vi "loadProg.vi"(11 "selected path":path) -> (0 "error out":errorcluster, 2 "scenes":T1[](array[typedef]), 3 "editArray":T2[](array[typedef]))   [LabVIEW 2014]
uses:
  typeDefs/editControl.ctl
  typeDefs/variantFlat.ctl
  typeDefs/pictChooser.ctl
  typeDefs/saveDataType.ctl
  <vilib>/picture/picture.llb/Draw True-Color Pixmap.vi
  <vilib>/Utility/config.llb/NI_LVConfig.lvlib
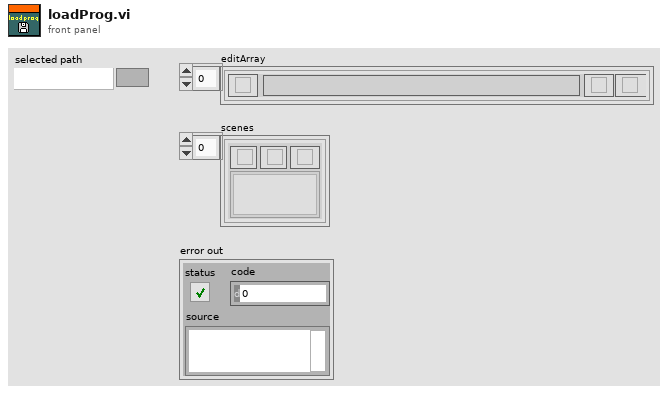
[diagram p1: front panel]
types:
  T1 = typedef "pictChooser.ctl" = cluster{"2D Picture":picture, "load":bool, "Path":path, "Bitmap":u32[][], "del":bool, "paint":bool}
  T2 = typedef "editControl.ctl" = cluster{"edit":bool, "info":string, "variantFlat":T3, "codeCluster":cluster{"code":u8[][]}, "del":bool, "ins":bool}
  T3 = typedef "variantFlat.ctl" = cluster{"type string":i16[], "data string":string}
  T4 = typedef "saveDataType.ctl" = cluster{"editArray":T2[], "bitmaps":cluster{"Bitmap":u32[][]}[], "paths":path[]}
  T5 = typedef "NI_LVConfig.lvlib/Config Data RefNum.ctl" = refnum<k1>
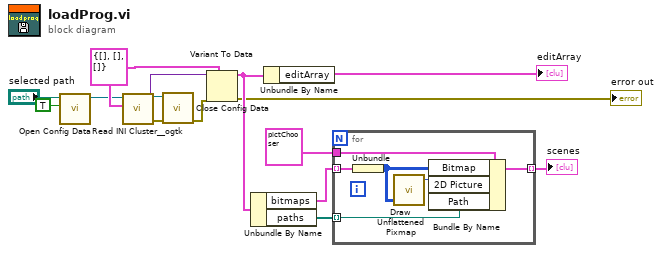
[diagram p0: block diagram]
diagram:
  w9 = T4 {"editArray"=[], "bitmaps"=[], "paths"=[]} ("saveData")
  n1 = call <vilib>:"Open Config Data.vi"("create file if necessary (T)"=TRUE, "configuration file path"="selected path") -> ("refnum"=w3:T5)  [unwired: 7 in, 2 out]
  n2 = call <userlib>:"Read INI Cluster__ogtk.vi"("INI Fomatted Cluster Type"=w9, "refnum"=w3) -> ("error out"=w4:errorcluster, "INI Fomatted Cluster"=w6:variant, "dup refnum"=w5:T5)  [unwired: 5 in, 2 out]
  n3 = call <vilib>:"Close Config Data.vi"("error in (no error)"=w4, "refnum"=w5) -> ("error out"=w7:errorcluster)  [unwired: 8 in, 1 out]
  n4 = Variant To Data(error in=w7, type=w9, Variant=w6) -> (data=w10:T4, error out=→"error out":errorcluster)
  n5 = Unbundle By Name(w10) -> ("bitmaps"=w11:cluster{"Bitmap":u32[][]}[], "paths"=w14:path[])
  n6 = Unbundle By Name(w10) -> ("editArray"=→"editArray":T2[])
  n7 = for {
    tunnel: w11 -> [w21] mode=indexing
    tunnel: T1 {"2D Picture"=bytes[0], "load"=FALSE, "Path"=path "", "Bitmap"=[], "del"=FALSE, "paint"=FALSE} ("pictChooser") -> [w20]
    tunnel: [w19] -> w13 mode=indexing
    tunnel: w14 -> [w16] mode=indexing
    n8 = Unbundle(w21) -> ("Bitmap"=w17:u32[][])
    n9 = call-poly <vilib>:"Draw Unflattened Pixmap.vi"("data (RGB format)"=w17) -> ("new picture"=w18:picture)  [unwired: 8 in]
    n10 = Bundle By Name(cluster=w20, "Bitmap"=w17, "2D Picture"=w18, "Path"=w16) -> (w19:T1)
  }
  "scenes" <- w13
